vi "Add To DAQmx Task.vi"(6 "Ignore Cal? (F)":bool, 7 "Voltage in":refnum<class "Voltage.lvclass">, 8 "error in (no error)":errorcluster, 9 "Scale Name":string, 10 "Chassis Name":string, 11 "task in":refnum<k21>) -> (0 "error out":errorcluster, 2 "Phys Chan Added":string, 3 "task out":refnum<k21>)   [LabVIEW 2012, in "Measurement Channels.lvlib" / "Voltage.lvclass"]
uses:
  Voltage.lvclass
  Voltage.lvclass/Voltage.ctl
  Class Channel/Read ChanName.vi
  Class Channel/Read Alias.vi
  Class Channel/Read Scale.vi
  Class Channel/Read Offset.vi
  Class Channel/Read Unit_EU.vi
  <vilib>/DAQmx/create/scale.llb/DAQmx Create Scale (Linear).vi
  <vilib>/DAQmx/create/channels.llb/DAQmx Create Channel (AI-Voltage-Basic).vi
  <resource>/objmgr/daqmx.rc
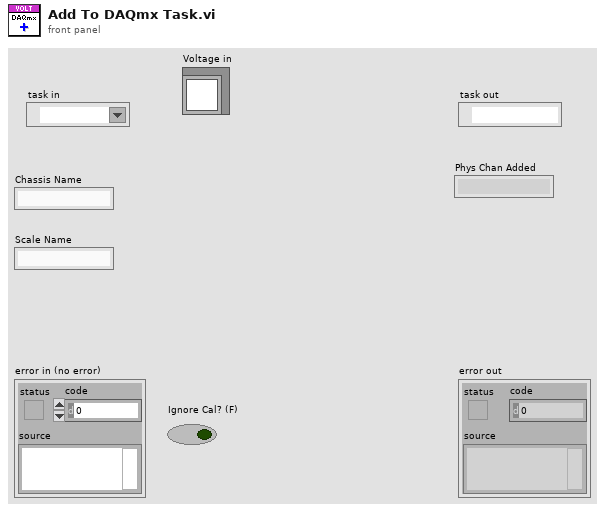
[diagram p1: front panel]
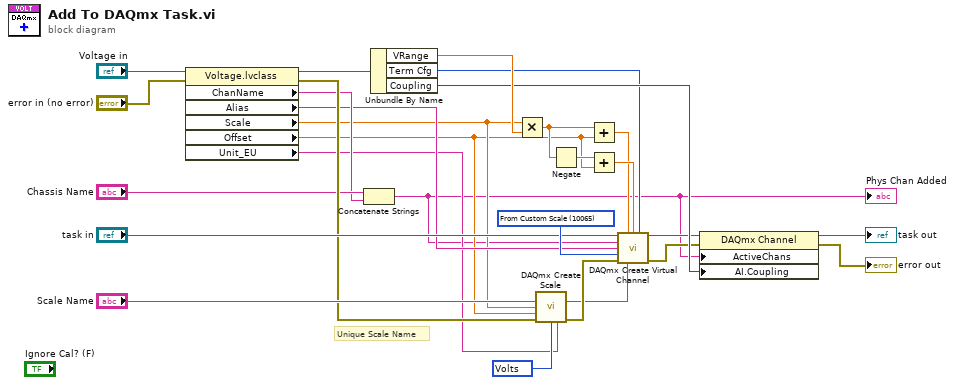
[diagram p0: block diagram]
diagram:
  w21 = 10348 items=["Volts"=10348, "Amps"=10342, "Deg F"=10144, "Deg C"=10143, "Deg R"=10145, "Kelvins"=10325, "Strain"=10299, "Ohms"=10384, "Hz"=10373, "Seconds"=10364, "Meters"=10219, "Inches"=10379, "Degrees"=10146, "Radians"=10273, "g"=10186, "m/s^2"=12470, "Pascals"=10081, "Newtons"=15875, "Pounds"=15876, "kgf"=15877, "psi"=15879, "bar"=15880, "Nm"=15881, "oz-in"=15882, "lb-in"=15883, "lb-ft"=15884, "Volts/Volt"=15896, "mVolts/Volt"=15897, "From TEDS"=12516] ("pre-scaled units")
  w17 = 10065 items=["Volts"=10348, "From Custom Scale"=10065] ("units")
  # "Unique Scale Name"
  n1 = property class="Voltage.lvclass"(reference="Voltage in", error in="error in (no error)") -> (reference out=w10:refnum<class "Voltage.lvclass">, error out=w8:errorcluster, "ChanName"=w6:string, "Alias"=w5:string, "Scale"=w4:dbl, "Offset"=w3:dbl, "Unit_EU"=w2:string)
  n2 = Concatenate Strings("Chassis Name", w6) -> (w1:string)
  "Phys Chan Added" <- w1
  n3 = Unbundle By Name(w10) -> ("VRange"=w24:dbl, "Term Cfg"=w16:u16, "Coupling"=w20:u16)
  n4 = Multiply(x=w4, y=w24) -> (x*y=w25:dbl)
  n5 = call-poly <vilib>:"DAQmx Create Scale.vi"("name"="Scale Name", "slope"=w4, "y-intercept"=w3, "error in"=w8, "pre-scaled units"=w21, "scaled units"=w2) -> ("scale out"=w22:tag, "error out"=w23:errorcluster)  [unwired: 8 in]
  n6 = Negate(x=w25) -> (-x=w26:dbl)
  n7 = Add(x=w25, y=w3) -> (x+y=w27:dbl)
  n8 = Add(x=w26, y=w3) -> (x+y=w28:dbl)
  n9 = call-poly <vilib>:"DAQmx Create Virtual Channel.vi"("task in"="task in", "maximum value"=w27, "minimum value"=w28, "input terminal configuration"=w16, "physical channels"=w1, "name to assign"=w5, "units"=w17, "error in"=w23, "custom scale name"=w22) -> ("task out"=w18:refnum<k21>, "error out"=w19:errorcluster)  [unwired: 5 in]
  n10 = property class="DAQmx Channel"(reference=w18, error in=w19, "ActiveChans"=w1, "AI.Coupling"=w20) -> (reference out=→"task out":refnum<k21>, error out=→"error out":errorcluster)
